vi "Code Recognition.vi"() -> ()   [LabVIEW 2020]
uses:
  <vilib>/Platform/TimedLoop/XDataNode/timing_clust.ctl
  <vilib>/Platform/TimedLoop/XDataNode/nitl_modes.ctl
  <vilib>/Platform/TimedLoop/XDataNode/wakeup.ctl
  <vilib>/Platform/TimedLoop/XDataNode/XDataNode.xnode
  <vilib>/High Genius/HG_Vision_Tookit/Functions/HG_CV.lvlib
  <vilib>/Platform/TimedLoop/XDataNode/XDNodeRunTimeDep.lvlib
panel:
  in  "stop":bool
  out "Identify Code Content":string
  out "Grayscale Image":picture
  # "Control Description:\n1. Gray Image: output 8-bit gray image.\n2. Identify Code Content: output the information identifying the QR code.\n\nProcedure Description:\n1. Running procedure.\n2. put the QR code into the camera field of view to identify the information."
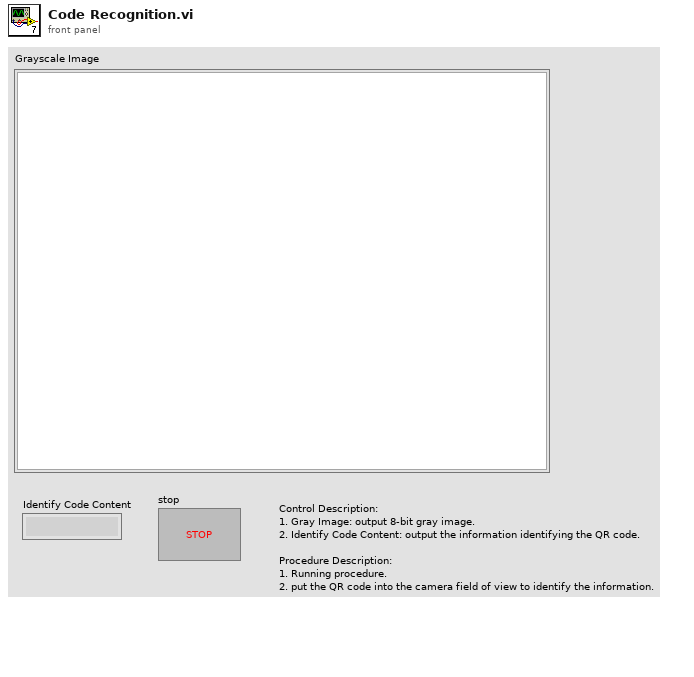
[diagram p1: front panel]
types:
  T1 = enum16{"320 (H)   x  240 (V)", "352(H)    x  288 (V)", "640 (H)   x  480 (V) ", "800 (H)   x  600 (V)", "1024 (H) x  768 (V)", "1280 (H) x  720 (V)", "1280 (H) x 1024 (V)", "1920 (H) x 1080 (V)"}
  T2 = enum16{"CV_8UC1", "CV_8SC1", "CV_16UC1", "CV_16SC1", "CV_32SC1", "CV_32FC1", "CV_64FC1", "7", "CV_8UC2", "CV_8SC2", "CV_16UC2", "CV_16SC2", "CV_32SC2", "CV_32FC2", "14", "16", "CV_8UC3", "CV_8SC3", "CV_16UC3", "CV_16SC3", "CV_32SC3", "CV_32FC3", "22", "23", "CV_8UC4", "CV_8SC4", "CV_16UC4", "CV_16SC4", "CV_32SC4", "CV_32FC4", "CV_64FC4", "31", "CV_8UC5", "CV_8SC5", "CV_16UC5", "CV_16SC5", "CV_32SC5", "CV_32FC5", "CV_64FC5", "39", "CV_8UC6", "CV_8SC6", "CV_16UC6", "CV_16SC6", "CV_32SC6", "CV_32FC6", "CV_64FC6"}
  T3 = typedef "XDNodeRunTimeDep.lvlib/timing_clust.ctl" = cluster{"Expected End [f-1]":u64, "Actual End [f-1]":u64, "Finished Late? [f-1]":bool, "Expected End [i-1]":u64, "Actual End [i-1]":u64, "Finished Late? [i-1]":bool, "Expected Start [i]":u64, "Actual Start [i]":u64, "Expected Start [f]":u64, "Actual Start [f]":u64, "Source Name":string, "Structure Name":string, "Period":i64, "Deadline":i64, "Offset":i64, "Start":i64, "Priority":i32, "Timeout":i32, "Mode":T4, "Wakeup Reason":T5, "Error":errorcluster, "Source Type":string, "Secondary Source Type":string, "Global End Time":u64, "Global Start Time":u64, "Frame Duration":u64, "Iteration Duration":u64, "Assigned CPU":i32, "I/O Scan Engine Mode":u32}
  T4 = typedef "XDNodeRunTimeDep.lvlib/nitl_modes.ctl" = enum32{"No Change", "Process missed periods, maintain original phase", "Discard missed periods, maintain original phase", "Process missed periods, ignore original phase", "Discard missed periods, ignore original phase"}
  T5 = typedef "XDNodeRunTimeDep.lvlib/wakeup.ctl" = enum32{"Normal", "Aborted", "Asynchronous wakeup", "Timing source error", "Timed loop error", "Timeout"}
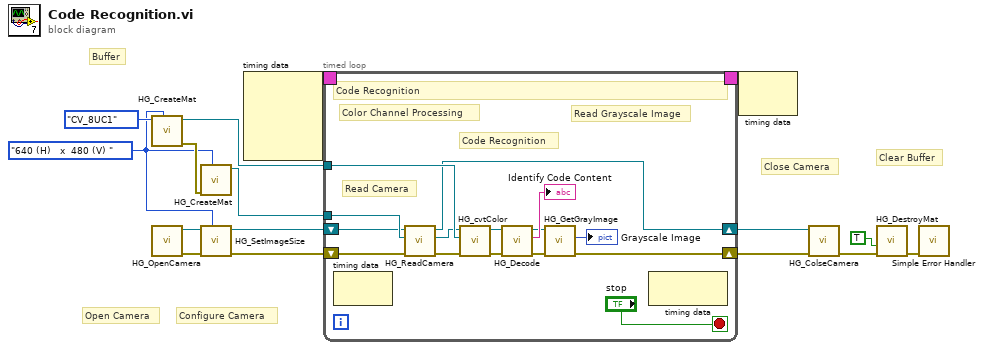
[diagram p0: block diagram]
diagram:
  w3 = T1."640 (H)   x  480 (V) " ("Image Size")
  # "Buffer"
  # "Clear Buffer"
  # "Close Camera"
  # "Configure Camera"
  # "Open Camera"
  n1 = call <vilib>:"HG_CreateMat.vi"("Image Size"=w3, "Type"=T2."CV_8UC1") -> ("error out"=w14:errorcluster, "Image Out"=w12:refnum<vi>)  [unwired: 8 in]
  n2 = call <vilib>:"HG_OpenCamera.vi"() -> ("error out"=w4:errorcluster, "IMAQ Session Out"=w10:refnum<k11>)  [unwired: 10 in]
  n3 = call <vilib>:"HG_CreateMat.vi"("Image Size"=w3, "error in (no error)"=w14) -> ("Image Out"=w8:refnum<vi>)  [unwired: 8 in, 1 out]
  n4 = call <vilib>:"HG_SetImageSize.vi"("Image Size"=w3, "error in (no error)"=w4, "IMAQ Session In"=w10) -> ("error out"=w5:errorcluster, "IMAQ Session Out"=w6:refnum<k11>)  [unwired: 7 in]
  n5 = node-c288() -> (w2:T3)  [unwired: 4 in]
  n6 = timed-loop {
    timing: w2 -> [_]
    timing-out: [_] -> w1
    tunnel: w12 -> [w31]
    tunnel: w8 -> [w29]
    shift-right: [w28] -> w7
    shift-left: w6 -> [w27]
    shift-right: [w30] -> w11
    shift-left: w5 -> [w26]
    stop <- "stop" stop-if-true
    # "Read Grayscale Image"
    # "Code Recognition"
    # "Color Channel Processing"
    # "Read Camera"
    # "Code Recognition"
    n7 = node-c288() -> ()  [unwired: 1 in, 1 out]
    n8 = call <vilib>:"HG_ReadCamera.vi"("error in (no error)"=w26, "Image In"=w29, "IMAQ Session In"=w27) -> ("error out"=w23:errorcluster, "Image Out"=w24:refnum<vi>, "IMAQ Session Out"=w28:refnum<k11>)  [unwired: 6 in]
    n9 = call <vilib>:"HG_cvtColor.vi"("error in (no error)"=w23, "Image Dst"=w31, "Image Src"=w24) -> ("error out"=w20:errorcluster, "Image Dst Out"=w21:refnum<vi>)  [unwired: 7 in]
    n10 = call <vilib>:"HG_Decode.vi"("error in (no error)"=w20, "Image In"=w21) -> ("error out"=w18:errorcluster, "string"=→"Identify Code Content":string, "Image Out"=w19:refnum<vi>)  [unwired: 7 in]
    n11 = call <vilib>:"HG_GetGrayImage.vi"("error in (no error)"=w18, "Image In"=w19) -> ("error out"=w30:errorcluster, "Picture"=→"Grayscale Image":picture)  [unwired: 7 in, 1 out]
    n12 = node-c288() -> ()  [unwired: 1 in, 1 out]
  }
  n13 = node-c288(w1) -> ()  [unwired: 1 out]
  n14 = call <vilib>:"HG_ColseCamera.vi"("error in (no error)"=w11, "IMAQ Session In"=w7) -> ("error out"=w9:errorcluster)  [unwired: 9 in]
  n15 = call <vilib>:"HG_DestroyMat.vi"("error in (no error)"=w9, "Boolean"=TRUE) -> ("error out"=w16:errorcluster)  [unwired: 8 in, 1 out]
  n16 = call <vilib>:"Simple Error Handler.vi"("error in (no error)"=w16) -> ()  [unwired: 4 in, 5 out]
